vi "Read Key Path.vi"(6 "Key Name":string, 7 "Section":string, 8 "error in (no error)":errorcluster, 10 "Section Element":variant, 11 "Path in":path) -> (0 "error out":errorcluster, 1 "found?":bool, 2 "Variant Element Data":variant, 3 "Path out":path, 4 "Key Name out":string)   [LabVIEW 2020, in "Generic Config Handling.lvlib"]
doc: "This vi reads a variant to a config file.\n\nIt only accepts very basic datatypes. \n\nIt will accept 1D and 2D arrays.\n\nIf key name is not wired, then it will use the name of the section element.\n\nSection Element in provides the type information and the default value."
uses:
  Generic Config Handling.lvlib
  <vilib>/Utility/config.llb/NI_LVConfig.lvlib
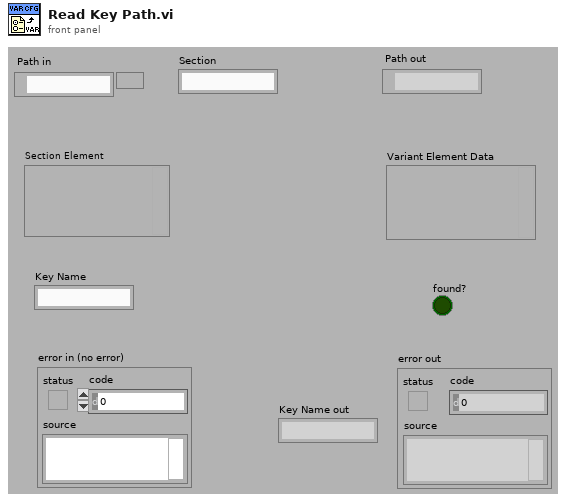
[diagram p1: front panel]
types:
  T1 = typedef "NI_LVConfig.lvlib/Config Data RefNum.ctl" = refnum<k1>
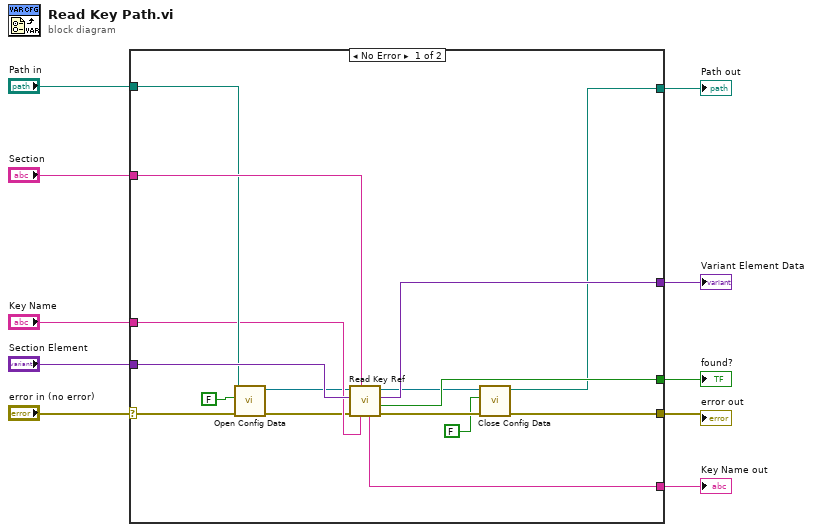
[diagram p0: block diagram]
diagram:
  n1 = case shown="No Error" "error in (no error)" {
    selector: "error in (no error)" -> [w11 w27]
    tunnel: [w26 _] -> w10
    tunnel: [w25 _] -> w9
    tunnel: [w24 w28] -> w8
    tunnel: "Section" -> [w23 _]
    tunnel: "Section Element" -> [w22 _]
    tunnel: "Path in" -> [w21 w29]
    tunnel: [w20 w29] -> w4
    tunnel: [w19 w27] -> w3
    tunnel: "Key Name" -> [w18 w28]
    frame No Error {
      n2 = call <vilib>:"Open Config Data.vi"("error in (no error)"=w11, "create file if necessary (T)"=FALSE, "configuration file path"=w21) -> ("error out"=w13:errorcluster, "refnum"=w14:T1)  [unwired: 6 in, 1 out]
      n3 = call "Read Key Ref.vi"("Key Name"=w18, "Section"=w23, "error in (no error)"=w13, "Section Element"=w22, "Refnum in"=w14) -> ("error out"=w16:errorcluster, "found?"=w25:bool, "Variant Element Data"=w26:variant, "Refnum out"=w17:T1, "Key Name out"=w24:string)  [unwired: 2 in]
      n4 = call <vilib>:"Close Config Data.vi"("error in (no error)"=w16, "write file if changed (T)"=FALSE, "refnum"=w17) -> ("error out"=w19:errorcluster, "file path"=w20:path)  [unwired: 7 in]
    }
    frame Error {
    }
  }
  "Path out" <- w4
  "error out" <- w3
  "Variant Element Data" <- w10
  "found?" <- w9
  "Key Name out" <- w8
